vi "Set OpMode.vi"(8 "error in (no error)":errorcluster, 11 "Value":u32(ring)=9 items=["位置"=8, "速度"=9, "扭矩"=10]) -> (0 "error out":errorcluster)   [LabVIEW 2020, in "输出轴伺服.lvlib"]
uses:
  Servo_global.vi
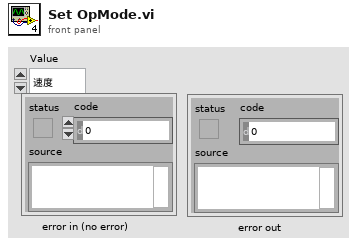
[diagram p1: front panel]
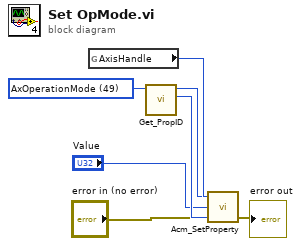
[diagram p0: block diagram]
diagram:
  w5 = u16 49 items=["AxTargetPosition"=44, "AxTargetVelocity"=45, "AxTargetTorque"=46, "AxControlWord"=47, "AxStatusWord"=48, "AxOperationMode"=49, "AxMaxTorque"=333] ("Prop")
  n1 = global read "Servo_global.vi" "AxisHandle"() -> (w7:u32)
  n2 = call "Get_PropID.vi"("Prop"=w5) -> ("BufferLength"=w4:u32, "PropID"=w6:u32)  [unwired: 9 in]
  n3 = call <userlib>:"Acm_SetProperty.vi"("Handle"=w7, "ProperyID"=w6, "Buffer"="Value", "Error Input(No Error)"="error in (no error)", "BufferLength"=w4) -> ("Error Output"=→"error out":errorcluster)  [unwired: 2 out]
